vi "exercise3.vi"() -> ()   [LabVIEW 2020]
uses:
  <vilib>/numeric/Random Number (Range) DBL.vi
panel:
  out "Phase Shift":dbl
  out "Cosine Graph":dbl[](graph)
  out "Sine Graph":dbl[](graph)
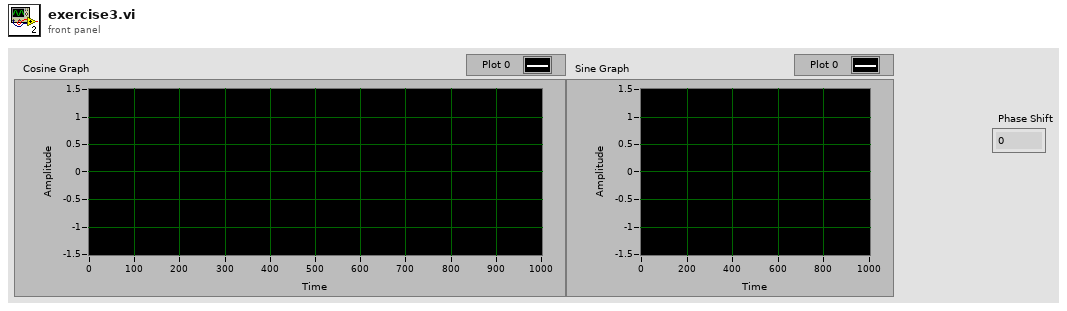
[diagram p1: front panel]
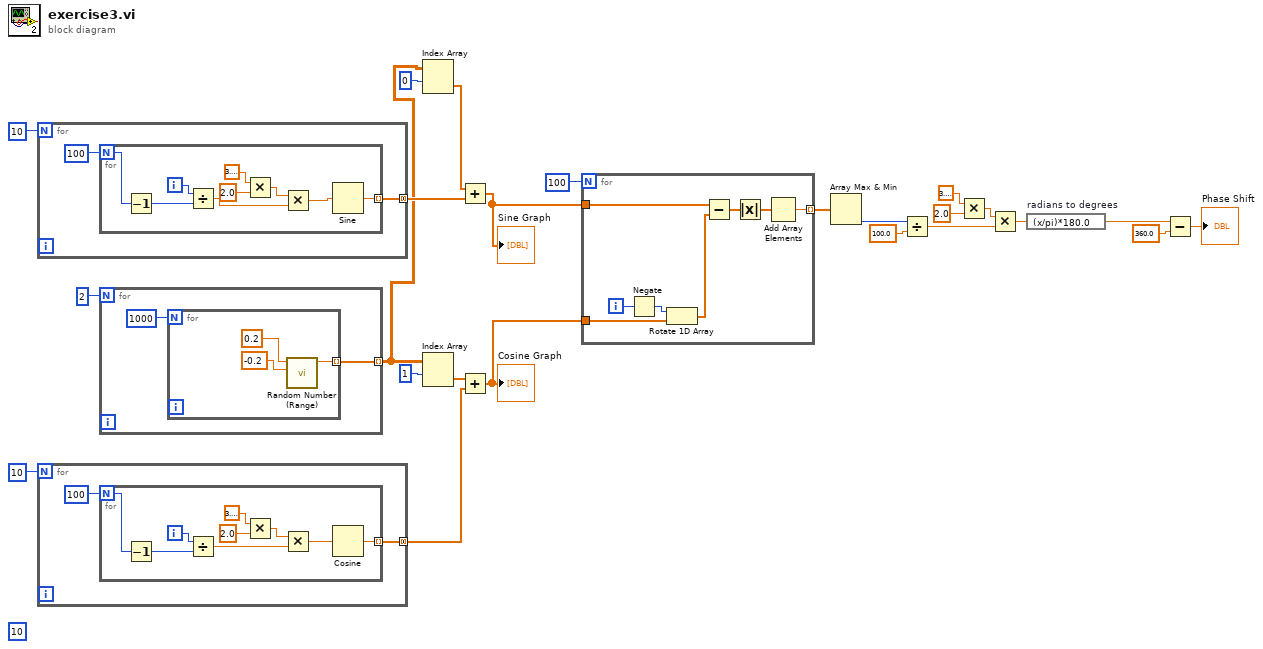
[diagram p0: block diagram]
diagram:
  (unwired) 10
  n1 = for {
    N: 10 -> [_]
    tunnel: [w25] -> w21 mode=concatenating
    n2 = for {
      N: 100 -> [w35]
      tunnel: [w30] -> w25 mode=indexing
      i -> [w28]
      n3 = Decrement(x=w35) -> (x-1=w27:i32)
      n4 = Divide(x=w28, y=w27) -> (x/y=w31:dbl)
      n5 = Multiply(x=3.141592653589793, y=2.0) -> (x*y=w32:dbl)
      n6 = Multiply(x=w32, y=w31) -> (x*y=w29:dbl)
      n7 = Sine(x=w29) -> (sin(x)=w30:dbl)
    }
  }
  n8 = for {
    N: 10 -> [_]
    tunnel: [w36] -> w16 mode=concatenating
    n9 = for {
      N: 100 -> [w46]
      tunnel: [w38] -> w36 mode=indexing
      i -> [w41]
      n10 = Decrement(x=w46) -> (x-1=w40:i32)
      n11 = Divide(x=w41, y=w40) -> (x/y=w42:dbl)
      n12 = Multiply(x=3.141592653589793, y=2.0) -> (x*y=w43:dbl)
      n13 = Multiply(x=w43, y=w42) -> (x*y=w39:dbl)
      n14 = Cosine(x=w39) -> (cos(x)=w38:dbl)
    }
  }
  n15 = for {
    N: 2 -> [_]
    tunnel: [w47] -> w17 mode=indexing
    n16 = for {
      N: 1000 -> [_]
      tunnel: [w49] -> w47 mode=indexing
      n17 = call-poly <vilib>:"Random Number (Range).vi"("lower bound (0)"=-0.2, "upper bound (100)"=0.2) -> ("number"=w49:dbl)  [unwired: 9 in]
    }
  }
  n18 = Index Array(array=w17, index (row)=0 ("index")) -> (element=w18:dbl[])  [unwired: 1 in]
  n19 = Index Array(array=w17, index (row)=1 ("index")) -> (element=w15:dbl[])  [unwired: 1 in]
  n20 = Add(x=w18, y=w21) -> (x+y=w14:dbl[])
  "Sine Graph" <- w14
  n21 = Add(x=w15, y=w16) -> (x+y=w13:dbl[])
  "Cosine Graph" <- w13
  n22 = for {
    N: 100 -> [_]
    tunnel: w14 -> [w59]
    tunnel: [w55] -> w11 mode=indexing
    tunnel: w13 -> [w57]
    i -> [w52]
    n23 = Negate(x=w52) -> (-x=w53:i32)
    n24 = Rotate 1D Array(1:w57, 2:w53) -> (0:w54:dbl[])
    n25 = Subtract(x=w59, y=w54) -> (x-y=w58:dbl[])
    n26 = Absolute Value(x=w58) -> (abs(x)=w56:dbl[])
    n27 = Add Array Elements(numeric array=w56) -> (sum=w55:dbl)
  }
  n28 = Array Max & Min(array=w11) -> (min index (indices)=w9:i32)  [unwired: 3 out]
  n29 = Divide(x=w9, y=100.0) -> (x/y=w8:dbl)
  n30 = Multiply(x=3.141592653589793, y=2.0) -> (x*y=w5:dbl)
  n31 = Multiply(x=w5, y=w8) -> (x*y=w4:dbl)
  n32 = expression code="(x/pi)*180.0" "radians to degrees"(w4) -> (w3:dbl)
  n33 = Subtract(x=w3, y=360.0) -> (x-y=→"Phase Shift":dbl)
